vi "Create Connection Configuration.vi"(8 "error in (no error)":errorcluster, 11 "Connection Configuration":T1) -> (0 "error out":errorcluster, 3 "SystemLink Configuration":refnum<class "NI Skyline Configuration.lvclass">)   [LabVIEW 2015, in "SystemLink File runtime.lvclass"]
doc: "Create SystemLink configuration based on configuration data in the DCAF configuration class.\n\nUse SystemLink's \"Close Configuration.vi\" to destroy configuration class after the SystemLink connection has been closed."
uses:
  SystemLink File runtime.lvclass
  configuration/Connection Configuration.ctl
  configuration/Connection Type.ctl
  <vilib>/Skyline/Configuration/Configuration_class/NI Skyline Configuration.lvclass
  <vilib>/Skyline/Configuration/Configuration AMQP_class/Open Configuration AMQP.vi
  <vilib>/Skyline/Configuration/Configuration HTTP_class/Open Configuration HTTP.vi
  <vilib>/Skyline/Configuration/Configuration HTTP_class/Open Configuration API Key.vi
  <vilib>/Skyline/Configuration/Configuration AMQP_class/NI Skyline Configuration AMQP.lvclass
  <vilib>/Skyline/Configuration/Configuration HTTP_class/NI Skyline Configuration HTTP.lvclass
  configuration/SystemLink File configuration.lvclass
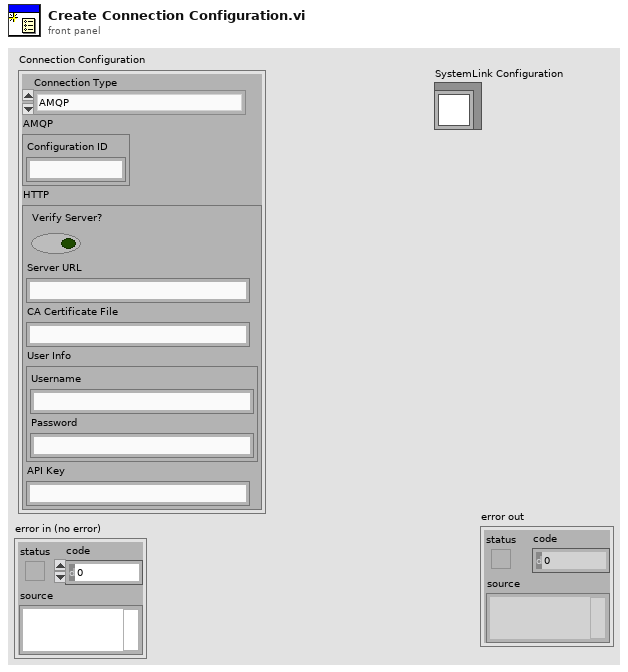
[diagram p1: front panel]
types:
  T1 = typedef "SystemLink File configuration.lvclass/Connection Configuration.ctl" = cluster{"Connection Type":T2, "AMQP":cluster{"Configuration ID":string}, "HTTP":cluster{"Verify Server?":bool, "Server URL":string, "CA Certificate File":string, "User Info":cluster{"Username":string, "Password":string}, "API Key":string}}
  T2 = typedef "SystemLink File configuration.lvclass/Connection Type.ctl" = enum16{"AMQP", "HTTP", "API Key (SystemLink Cloud)"}
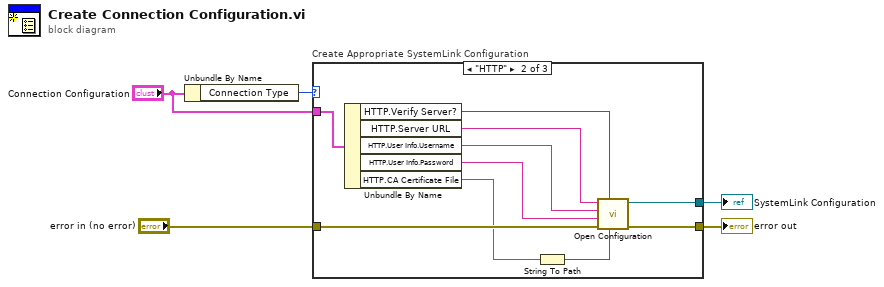
[diagram p0: block diagram]
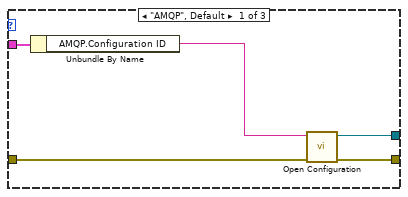
[diagram p2: hidden frame]
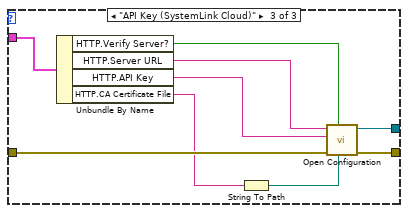
[diagram p3: hidden frame]
diagram:
  n1 = Unbundle By Name("Connection Configuration") -> ("Connection Type"=w3:T2)
  n2 = case "Create Appropriate SystemLink Configuration" shown="\"HTTP\"" w3 {
    tunnel: "error in (no error)" -> [w10 w19 w27]
    tunnel: [w9 w20 w28] -> w4
    tunnel: "Connection Configuration" -> [w7 w17 w26]
    tunnel: [w8 w18 w29] -> w1
    frame "AMQP", Default {
      n3 = Unbundle By Name(w7) -> ("AMQP.Configuration ID"=w6:string)
      n4 = call-poly <vilib>:"Open Configuration.vi"("error in (no error)"=w10, "configuration id"=w6) -> ("error out"=w9:errorcluster, "AMQP configuration out"=w8:refnum<class "NI Skyline Configuration AMQP.lvclass">)  [unwired: 8 in]
    }
    frame "HTTP" {
      n5 = Unbundle By Name(w17) -> ("HTTP.Verify Server?"=w16:bool, "HTTP.Server URL"=w15:string, "HTTP.User Info.Username"=w14:string, "HTTP.User Info.Password"=w13:string, "HTTP.CA Certificate File"=w11:string)
      n6 = String To Path(string=w11) -> (path=w12:path)
      n7 = call-poly <vilib>:"Open Configuration.vi"("ca certificate file"=w12, "verify server?"=w16, "error in (no error)"=w19, "password"=w13, "username"=w14, "server url"=w15) -> ("error out"=w20:errorcluster, "HTTP configuration out"=w18:refnum<class "NI Skyline Configuration HTTP.lvclass">)  [unwired: 4 in]
    }
    frame "API Key (SystemLink Cloud)" {
      n8 = Unbundle By Name(w26) -> ("HTTP.Verify Server?"=w25:bool, "HTTP.Server URL"=w24:string, "HTTP.API Key"=w23:string, "HTTP.CA Certificate File"=w21:string)
      n9 = String To Path(string=w21) -> (path=w22:path)
      n10 = call-poly <vilib>:"Open Configuration.vi"("ca certificate file"=w22, "verify server?"=w25, "error in (no error)"=w27, "api key"=w23, "server url"=w24) -> ("error out"=w28:errorcluster, "HTTP configuration out"=w29:refnum<class "NI Skyline Configuration HTTP.lvclass">)  [unwired: 5 in]
    }
  }
  "error out" <- w4
  "SystemLink Configuration" <- w1
